vi "GetAccTimes.vi"(8 "错误输入（无错误）":errorcluster) -> (0 "错误输出":errorcluster, 3 "采样缓存区累积采样数据次数":u8)   [LabVIEW 2014]
uses:
  X86Dll/ZXUTConfigMgr.dll
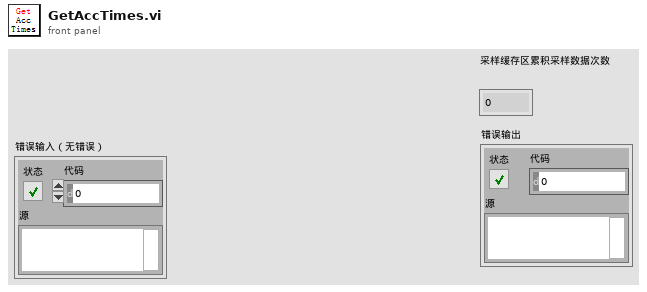
[diagram p1: front panel]
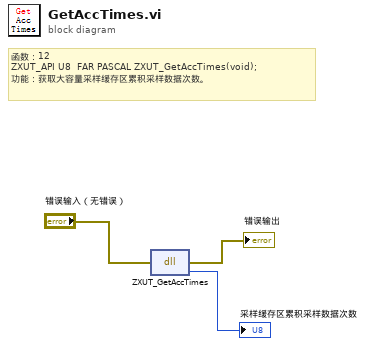
[diagram p0: block diagram]
diagram:
  # "函数：12\nZXUT_API U8\t\tFAR PASCAL ZXUT_GetAccTimes(void);\n功能：获取大容量采样缓存区累积采样数据次数。"
  n1 = dll-call lib="D:/Software/Utrasonic on-line monitoring/X86Dll/ZXUTConfigMgr.dll" fn="ZXUT_GetAccTimes"(error in="错误输入（无错误）") -> (error out=→"错误输出":errorcluster, "返回类型"=→"采样缓存区累积采样数据次数":u8)  [unwired: 2 in, 1 out]
